vi "PulseParseParams.vi"(2 "Pars cluster":T1, 3 "Pars String":string) -> (0 "Recompile each run?":bool, 1 "Pars cluster":T1)   [LabVIEW 2017]
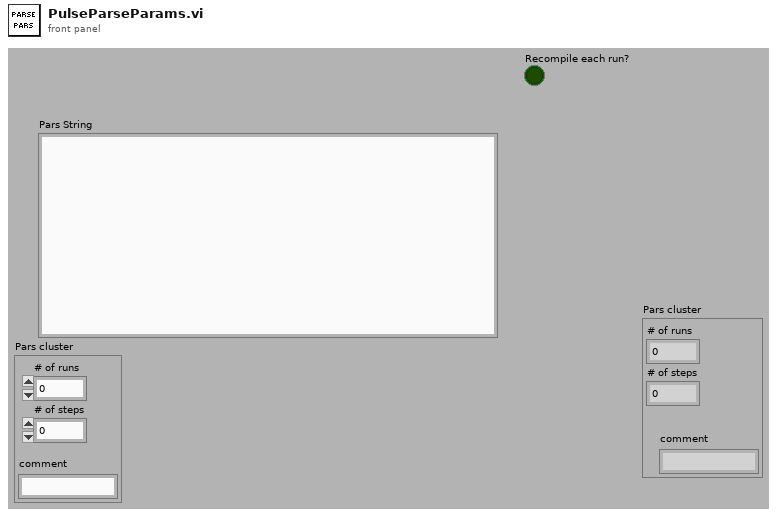
[diagram p1: front panel]
types:
  T1 = cluster{"# of runs":i32, "# of steps":i32, "comment":string}
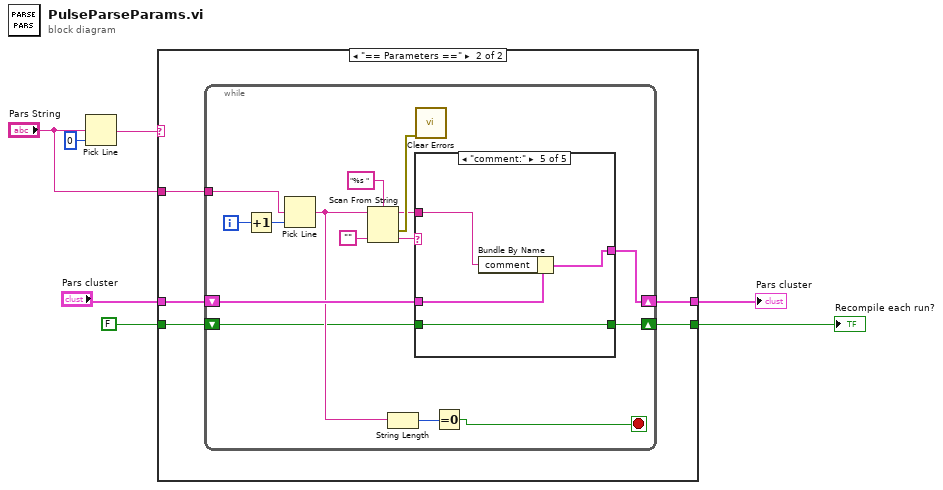
[diagram p0: block diagram]
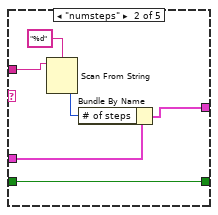
[diagram p4: hidden frame]
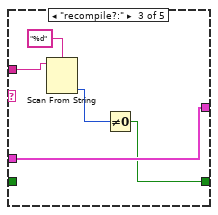
[diagram p5: hidden frame]
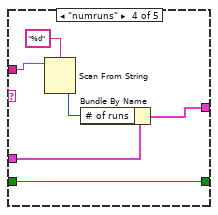
[diagram p6: hidden frame]
diagram:
  n1 = Pick Line(multi-line string="Pars String", line index=0) -> (output string=w6:string)  [unwired: 1 in]
  n2 = case shown="\"== Parameters ==\"" w6 {
    tunnel: "Pars cluster" -> [w9 w14]
    tunnel: [w9 w13] -> w3
    tunnel: "Pars String" -> [_ w12]
    tunnel: FALSE -> [w8 w11]
    tunnel: [w8 w10] -> w1
    frame "False", Default {
    }
    frame "== Parameters ==" {
      n3 = while {
        shift-right: [w23] -> w13
        shift-left: w14 -> [w24]
        tunnel: w12 -> [w22]
        shift-right: [w15] -> w10
        shift-left: w11 -> [w16]
        i -> [w28]
        stop <- w19 stop-if-true
        n4 = Increment(x=w28) -> (x+1=w29:i32)
        n5 = Pick Line(multi-line string=w22, line index=w29) -> (output string=w21:string)  [unwired: 1 in]
        n6 = Scan From String(format string="%s ", input string=w21, default 1="") -> (remaining string=w17:string, error out=w18:errorcluster, output 1=w25:string)  [unwired: 2 in, 1 out]
        n7 = String Length(string=w21) -> (length=w20:i32)
        n8 = case shown="\"comment:\"" w25 {
          tunnel: w24 -> [w31 w37 w40 w47 w52]
          tunnel: [w31 w36 w40 w48 w51] -> w23
          tunnel: w17 -> [_ w35 w42 w45 w50]
          tunnel: w16 -> [w30 w32 _ w43 w49]
          tunnel: [w30 w32 w38 w43 w49] -> w15
          frame "False", Default {
          }
          frame "numsteps" {
            n9 = Scan From String(format string="%d", input string=w35) -> (output 1=w33:i32)  [unwired: 3 in, 3 out]
            n10 = Bundle By Name(cluster=w37, "# of steps"=w33) -> (w36:T1)
          }
          frame "recompile?:" {
            n11 = Scan From String(format string="%d", input string=w42) -> (output 1=w39:i32)  [unwired: 3 in, 3 out]
            n12 = Not Equal To 0?(x=w39) -> (x != 0?=w38:bool)
          }
          frame "numruns" {
            n13 = Scan From String(format string="%d", input string=w45) -> (output 1=w44:i32)  [unwired: 3 in, 3 out]
            n14 = Bundle By Name(cluster=w47, "# of runs"=w44) -> (w48:T1)
          }
          frame "comment:" {
            n15 = Bundle By Name(cluster=w52, "comment"=w50) -> (w51:T1)
          }
        }
        n16 = call <vilib>:"Clear Errors.vi"("error in (no error)"=w18) -> ()  [unwired: 5 in, 2 out]
        n17 = Equal To 0?(x=w20) -> (x = 0?=w19:bool)
      }
    }
  }
  "Pars cluster" <- w3
  "Recompile each run?" <- w1
